vi "Func-엑셀 데이터를 그래프로 출력.vi"() -> ()   [LabVIEW 2015] (continued)
586.53\n586.54\n586.56\n586.58\n586.59\n586.61\n586.63\n586.64\n586.66\n586.68\n586.69\n586.71\n586.73\n586.74\n586.76\n586.78\n586.79\n586.81\n586.83\n586.84\n586.86\n586.88\n586.89\n586.91\n586.93\n586.95\n586.96\n586.98\n586.99\n587.01\n587.03\n587.04\n587.06\n587.08\n587.09\n587.11\n587.13\n587.14\n587.16\n587.18\n587.19\n587.21\n587.23\n587.24\n587.26\n587.28\n587.29\n587.31\n587.33\n587.34\n587.36\n587.38\n587.39\n587.41\n587.43\n587.44\n587.46\n587.48\n587.49\n587.51\n587.53\n587.54\n587.56\n587.58\n587.59\n587.61\n587.63\n587.65\n587.66\n587.68\n587.69\n587.71\n587.73\n587.74\n587.76\n587.78\n587.79\n587.81\n587.83\n587.84\n587.86\n587.88\n587.89\n587.91\n587.93\n587.94\n587.96\n587.98\n587.99\n588.01\n588.03\n588.04\n588.06\n588.08\n588.09\n588.11\n588.13\n588.14\n588.16\n588.18\n588.19\n588.21\n588.23\n588.24\n588.26\n588.28\n588.29\n588.31\n588.33\n588.34\n588.36\n588.38\n588.39\n588.41\n588.43\n588.44\n588.46\n588.48\n588.49\n588.51\n588.53\n588.54\n588.56\n588.58\n588.59\n588.61\n588.63\n588.64\n588.66\n588.68\n588.69\n588.71\n588.73\n588.74\n588.76\n588.78\n588.79\n588.81\n588.83\n588.84\n588.86\n588.88\n588.89\n588.91\n588.93\n588.94\n588.96\n588.98\n589\n589.01\n589.03\n589.04\n589.06\n589.08\n589.09\n589.11\n589.13\n589.14\n589.16\n589.18\n589.19\n589.21\n589.23\n589.24\n589.26\n589.28\n589.29\n589.31\n589.33\n589.35\n589.36\n589.38\n589.39\n589.41\n589.43\n589.45\n589.46\n589.48\n589.49\n589.51\n589.53\n589.54\n589.56\n589.58\n589.6\n589.61\n589.63\n589.64\n589.66\n589.68\n589.69\n589.71\n589.73\n589.74\n589.76\n589.78\n589.79\n589.81\n589.83\n589.84\n589.86\n589.88\n589.89\n589.91\n589.93\n589.94\n589.96\n589.98\n589.99\n590.01\n590.03\n590.04\n590.06\n590.08\n590.09\n590.11\n590.13\n590.15\n590.16\n590.18\n590.19\n590.21\n590.23\n590.24\n590.26\n590.28\n590.29\n590.31\n590.33\n590.34\n590.36\n590.38\n590.39\n590.41\n590.43\n590.44\n590.46\n590.48\n590.5\n590.51\n590.53\n590.54\n590.56\n590.58\n590.59\n590.61\n590.63\n590.64\n590.66\n590.68\n590.69\n590.71\n590.73\n590.74\n590.76\n590.78\n590.79\n590.81\n590.83\n590.84\n590.86\n590.88\n590.89\n590.91\n590.93\n590.94\n590.96\n590.98\n590.99\n591.01\n591.03\n591.04\n591.06\n591.08\n591.09\n591.11\n591.13\n591.14\n591.16\n591.18\n591.19\n591.21\n591.23\n591.24\n591.26\n591.28\n591.29\n591.31\n591.33\n591.34\n591.36\n591.38\n591.39\n591.41\n591.43\n591.44\n591.46\n591.48\n591.49\n591.51\n591.53\n591.54\n591.56\n591.58\n591.59\n591.61\n591.63\n591.64\n591.66\n591.68\n591.69\n591.71\n591.73\n591.75\n591.76\n591.78\n591.79\n591.81\n591.83\n591.84\n591.86\n591.88\n591.89\n591.91\n591.93\n591.94\n591.96\n591.98\n591.99\n592.01\n592.03\n592.04\n592.06\n592.08\n592.1\n592.11\n592.13\n592.14\n592.16\n592.18\n592.19\n592.21\n592.23\n592.24\n592.26\n592.28\n592.29\n592.31\n592.33\n592.34\n592.36\n592.38\n592.39\n592.41\n592.43\n592.45\n592.46\n592.48\n592.49\n592.51\n592.53\n592.54\n592.56\n592.58\n592.59\n592.61\n592.63\n592.64\n592.66\n592.68\n592.7\n592.71\n592.73\n592.74\n592.76\n592.78\n592.8\n592.81\n592.83\n592.84\n592.86\n592.88\n592.89\n592.91\n592.93\n592.94\n592.96\n592.98\n592.99\n593.01\n593.03\n593.05\n593.06\n593.08\n593.09\n593.11\n593.13\n593.15\n593.16\n593.18\n593.19\n593.21\n593.23\n593.25\n593.26\n593.28\n593.29\n593.31\n593.33\n593.34\n593.36\n593.38\n593.39\n593.41\n593.43\n593.44\n593.46\n593.48\n593.49\n593.51\n593.53\n593.54\n593.56\n593.58\n593.59\n593.61\n593.63\n593.65\n593.66\n593.68\n593.69\n593.71\n593.73\n593.75\n593.76\n593.78\n593.79\n593.81\n593.83\n593.84\n593.86\n593.88\n593.89\n593.91\n593.93\n593.94\n593.96\n593.98\n593.99\n594.01\n594.03\n594.04\n594.06\n594.08\n594.09\n594.11\n594.13\n594.14\n594.16\n594.18\n594.19\n594.21\n594.23\n594.24\n594.26\n594.28\n594.29\n594.31\n594.33\n594.34\n594.36\n594.38\n594.39\n594.41\n594.43\n594.44\n594.46\n594.48\n594.49\n594.51\n594.53\n594.54\n594.56\n594.58\n594.59\n594.61\n594.63\n594.64\n594.66\n594.68\n594.69\n594.71\n594.73\n594.74\n594.76\n594.78\n594.79\n594.81\n594.83\n594.85\n594.86\n594.88\n594.89\n594.91\n594.93\n594.94\n594.96\n594.98\n594.99\n595.01\n595.03\n595.04\n595.06\n595.08\n595.09\n595.11\n595.13\n595.14\n595.16\n595.18\n595.2\n595.21\n595.23\n595.24\n595.26\n595.28\n595.29\n595.31\n595.33\n595.34\n595.36\n595.38\n595.39\n595.41\n595.43\n595.45\n595.46\n595.48\n595.49\n595.51\n595.53\n595.55\n595.56\n595.58\n595.59\n595.61\n595.63\n595.64\n595.66\n595.68\n595.69\n595.71\n595.73\n595.74\n595.76\n595.78\n595.8\n595.81\n595.83\n595.84\n595.86\n595.88\n595.89\n595.91\n595.93\n595.94\n595.96\n595.98\n595.99\n596.01\n596.03\n596.04\n596.06\n596.08\n596.09\n596.11\n596.13\n596.14\n596.16\n596.18\n596.19\n596.21\n596.23\n596.24\n596.26\n596.28\n596.29\n596.31\n596.33\n596.34\n596.36\n596.38\n596.39\n596.41\n596.43\n596.44\n596.46\n596.48\n596.5\n596.51\n596.53\n596.54\n596.56\n596.58\n596.6\n596.61\n596.63\n596.64\n596.66\n596.68\n596.7\n596.71\n596.73\n596.74\n596.76\n596.78\n596.79\n596.81\n596.83\n596.84\n596.86\n596.88\n596.89\n596.91\n596.93\n596.94\n596.96\n596.98\n596.99\n597.01\n597.03\n597.04\n597.06\n597.08\n597.09\n597.11\n597.13\n597.14\n597.16\n597.18\n597.19\n597.21\n597.23\n597.24\n597.26\n597.28\n597.29\n597.31\n597.33\n597.34\n597.36\n597.38\n597.39\n597.41\n597.43\n597.44\n597.46\n597.48\n597.49\n597.51\n597.53\n597.54\n597.56\n597.58\n597.59\n597.61\n597.63\n597.64\n597.66\n597.68\n597.69\n597.71\n597.73\n597.74\n597.76\n597.78\n597.79\n597.81\n597.83\n597.84\n597.86\n597.88\n597.89\n597.91\n597.93\n597.94\n597.96\n597.98\n597.99\n598.01\n598.03\n598.04\n598.06\n598.08\n598.09\n598.11\n598.13\n598.14\n598.16\n598.18\n598.2\n598.21\n598.23\n598.24\n598.26\n598.28\n598.29\n598.31\n598.33\n598.34\n598.36\n598.38\n598.39\n598.41\n598.43\n598.44\n598.46\n598.48\n598.49\n598.51\n598.53\n598.55\n598.56\n598.58\n598.59\n598.61\n598.63\n598.65\n598.66\n598.68\n598.69\n598.71\n598.73\n598.74\n598.76\n598.78\n598.8\n598.81\n598.83\n598.84\n598.86\n598.88\n598.9\n598.91\n598.93\n598.94\n598.96\n598.98\n599\n599.01\n599.03\n599.04\n599.06\n599.08\n599.09\n599.11\n599.13\n599.14\n599.16\n599.18\n599.19\n599.21\n599.23\n599.25\n599.26\n599.28\n599.29\n599.31\n599.33\n599.34\n599.36\n599.38\n599.39\n599.41\n599.43\n599.44\n599.46\n599.48\n599.49\n599.51\n599.53\n599.54\n599.56\n599.58\n599.59\n599.61\n599.63\n599.64\n599.66\n599.68\n599.69\n599.71\n599.73\n599.75\n599.76\n599.78\n599.79\n599.81\n599.83\n599.84\n599.86\n599.88\n599.89\n599.91\n599.93\n599.94\n599.96\n599.98\n599.99\n600.01\n600.03\n600.04\n600.06\n600.08\n600.09\n600.11\n600.13\n600.14\n600.16\n600.18\n600.19\n600.21\n600.23\n600.24\n600.26\n600.28\n600.29\n600.31\n600.33\n600.34\n600.36\n600.38\n600.39\n600.41\n600.43\n600.44\n600.46\n600.48\n600.49\n600.51\n600.53\n600.54\n600.56\n600.58\n600.59\n600.61\n600.63\n600.64\n600.66\n600.68\n600.69\n600.71\n600.73\n600.74\n600.76\n600.78\n600.79\n600.81\n600.83\n600.84\n600.86\n600.88\n600.89\n600.91\n600.93\n600.94\n600.96\n600.98\n600.99\n601.01\n601.03\n601.04\n601.06\n601.08\n601.09\n601.11\n601.13\n601.14\n601.16\n601.18\n601.19\n601.21\n601.23\n601.24\n601.26\n601.28\n601.3\n601.31\n601.33\n601.34\n601.36\n601.38\n601.39\n601.41\n601.43\n601.44\n601.46\n601.48\n601.49\n601.51\n601.53\n601.54\n601.56\n601.58\n601.59\n601.61\n601.63\n601.65\n601.66\n601.68\n601.69\n601.71\n601.73\n601.75\n601.76\n601.78\n601.79\n601.81\n601.83\n601.84\n601.86\n601.88\n601.9\n601.91\n601.93\n601.94\n601.96\n601.98\n602\n602.01\n602.03\n602.04\n602.06\n602.08\n602.09\n602.11\n602.13\n602.14\n602.16\n602.18\n602.19\n602.21\n602.23\n602.25\n602.26\n602.28\n602.29\n602.31\n602.33\n602.34\n602.36\n602.38\n602.39\n602.41\n602.43\n602.44\n602.46\n602.48\n602.49\n602.51\n602.53\n602.54\n602.56\n602.58\n602.6\n602.61\n602.63\n602.64\n602.66\n602.68\n602.69\n602.71\n602.73\n602.74\n602.76\n602.78\n602.79\n602.81\n602.83\n602.84\n602.86\n602.88\n602.89\n602.91\n602.93\n602.94\n602.96\n602.98\n602.99\n603.01\n603.03\n603.04\n603.06\n603.08\n603.09\n603.11\n603.13\n603.14\n603.16\n603.18\n603.19\n603.21\n603.23\n603.24\n603.26\n603.28\n603.29\n603.31\n603.33\n603.34\n603.36\n603.38\n603.39\n603.41\n603.43\n603.44\n603.46\n603.48\n603.49\n603.51\n603.53\n603.54\n603.56\n603.58\n603.59\n603.61\n603.63\n603.64\n603.66\n603.68\n603.69\n603.71\n603.73\n603.74\n603.76\n603.78\n603.79\n603.81\n603.83\n603.84\n603.86\n603.88\n603.89\n603.91\n603.93\n603.94\n603.96\n603.98\n603.99\n604.01\n604.03\n604.04\n604.06\n604.08\n604.09\n604.11\n604.13\n604.14\n604.16\n604.18\n604.19\n604.21\n604.23\n604.24\n604.26\n604.28\n604.29\n604.31\n604.33\n604.34\n604.36\n604.38\n604.4\n604.41\n604.43\n604.44\n604.46\n604.48\n604.49\n604.51\n604.53\n604.54\n604.56\n604.58\n604.59\n604.61\n604.63\n604.64\n604.66\n604.68\n604.69\n604.71\n604.73\n604.75\n604.76\n604.78\n604.79\n604.81\n604.83\n604.85\n604.86\n604.88\n604.89\n604.91\n604.93\n604.94\n604.96\n604.98\n605\n605.01\n605.03\n605.04\n605.06\n605.08\n605.1\n605.11\n605.13\n605.14\n605.16\n605.18\n605.19\n605.21\n605.23\n605.24\n605.26\n605.28\n605.29\n605.31\n605.33\n605.34\n605.36\n605.38\n605.39\n605.41\n605.43\n605.44\n605.46\n605.48\n605.49\n605.51\n605.53\n605.55\n605.56\n605.58\n605.59\n605.61\n605.63\n605.64\n605.66\n605.68\n605.69\n605.71\n605.73\n605.74\n605.76\n605.78\n605.8\n605.81\n605.83\n605.84\n605.86\n605.88\n605.89\n605.91\n605.93\n605.94\n605.96\n605.98\n605.99\n606.01\n606.03\n606.04\n606.06\n606.08\n606.09\n606.11\n606.13\n606.14\n606.16\n606.18\n606.19\n606.21\n606.23\n606.24\n606.26\n606.28\n606.29\n606.31\n606.33\n606.34\n606.36\n606.38\n606.39\n606.41\n606.43\n606.44\n606.46\n606.48\n606.49\n606.51\n606.53\n606.54\n606.56\n606.58\n606.59\n606.61\n606.63\n606.64\n606.66\n606.68\n606.69\n606.71\n606.73\n606.74\n606.76\n606.78\n606.79\n606.81\n606.83\n606.84\n606.86\n606.88\n606.89\n606.91\n606.93\n606.94\n606.96\n606.98\n606.99\n607.01\n607.03\n607.04\n607.06\n607.08\n607.09\n607.11\n607.13\n607.14\n607.16\n607.18\n607.19\n607.21\n607.23\n607.24\n607.26\n607.28\n607.29\n607.31\n607.33\n607.34\n607.36\n607.38\n607.39\n607.41\n607.43\n607.44\n607.46\n607.48\n607.5\n607.51\n607.53\n607.54\n607.56\n607.58\n607.59\n607.61\n607.63\n607.64\n607.66\n607.68\n607.69\n607.71\n607.73\n607.75\n607.76\n607.78\n607.79\n607.81\n607.83\n607.85\n607.86\n607.88\n607.89\n607.91\n607.93\n607.94\n607.96\n607.98\n607.99\n608.01\n608.03\n608.04\n608.06\n608.08\n608.09\n608.11\n608.13\n608.14\n608.16\n608.18\n608.19\n608.21\n608.23\n608.24\n608.26\n608.28\n608.29\n608.31\n608.33\n608.34\n608.36\n608.38\n608.39\n608.41\n608.43\n608.44\n608.46\n608.48\n608.49\n608.51\n608.53\n608.55\n608.56\n608.58\n608.59\n608.61\n608.63\n608.64\n608.66\n608.68\n608.69\n608.71\n608.73\n608.74\n608.76\n608.78\n608.8\n608.81\n608.83\n608.84\n608.86\n608.88\n608.89\n608.91\n608.93\n608.94\n608.96\n608.98\n608.99\n609.01\n609.03\n609.04\n609.06\n609.08\n609.09\n609.11\n609.13\n609.14\n609.16\n609.18\n609.19\n609.21\n609.23\n609.24\n609.26\n609.28\n609.29\n609.31\n609.33\n609.34\n609.36\n609.38\n609.39\n609.41\n609.43\n609.44\n609.46\n609.48\n609.49\n609.51\n609.53\n609.54\n609.56\n609.58\n609.59\n609.61\n609.63\n609.64\n609.66\n609.68\n609.69\n609.71\n609.73\n609.74\n609.76\n609.78\n609.79\n609.81\n609.83\n609.84\n609.86\n609.88\n609.89\n609.91\n609.93\n609.94\n609.96\n609.98\n609.99\n610.01\n610.03\n610.04\n610.06\n610.08\n610.09\n610.11\n610.13\n610.14\n610.16\n610.18\n610.19\n610.21\n610.23\n610.24\n610.26\n610.28\n610.29\n610.31\n610.33\n610.34\n610.36\n610.38\n610.39\n610.41\n610.43\n610.44\n610.46\n610.48\n610.5\n610.51\n610.53\n610.54\n610.56\n610.58\n610.6\n610.61\n610.63\n610.64\n610.66\n610.68\n610.69\n610.71\n610.73\n610.74\n610.76\n610.78\n610.79\n610.81\n610.83\n610.85\n610.86\n610.88\n610.89\n610.91\n610.93\n610.95\n610.96\n610.98\n610.99\n611.01\n611.03\n611.04\n611.06\n611.08\n611.1\n611.11\n611.13\n611.14\n611.16\n611.18\n611.2\n611.21\n611.23\n611.24\n611.26\n611.28\n611.3\n611.31\n611.33\n611.34\n611.36\n611.38\n611.39\n611.41\n611.43\n611.44\n611.46\n611.48\n611.49\n611.51\n611.53\n611.54\n611.56\n611.58\n611.59\n611.61\n611.63\n611.64\n611.66\n611.68\n611.69\n611.71\n611.73\n611.74\n611.76\n611.78\n611.79\n611.81\n611.83\n611.84\n611.86\n611.88\n611.89\n611.91\n611.93\n611.94\n611.96\n611.98\n611.99\n612.01\n612.03\n612.04\n612.06\n612.08\n612.09\n612.11\n612.13\n612.14\n612.16\n612.18\n612.19\n612.21\n612.23\n612.24\n612.26\n612.28\n612.29\n612.31\n612.33\n612.35\n612.36\n612.38\n612.39\n612.41\n612.43\n612.44\n612.46\n612.48\n612.49\n612.51\n612.53\n612.54\n612.56\n612.58\n612.59\n612.61\n612.63\n612.64\n612.66\n612.68\n612.69\n612.71\n612.73\n612.74\n612.76\n612.78\n612.79\n612.81\n612.83\n612.84\n612.86\n612.88\n612.89\n612.91\n612.93\n612.94\n612.96\n612.98\n612.99\n613.01\n613.03\n613.04\n613.06\n613.08\n613.09\n613.11\n613.13\n613.14\n613.16\n613.18\n613.19\n613.21\n613.23\n613.24\n613.26\n613.28\n613.29\n613.31\n613.33\n613.34\n613.36\n613.38\n613.39\n613.41\n613.43\n613.44\n613.46\n613.48\n613.49\n613.51\n613.53\n613.54\n613.56\n613.58\n613.6\n613.61\n613.63\n613.64\n613.66\n613.68\n613.69\n613.71\n613.73\n613.74\n613.76\n613.78\n613.79\n613.81\n613.83\n613.84\n613.86\n613.88\n613.89\n613.91\n613.93\n613.95\n613.96\n613.98\n613.99\n614.01\n614.03\n614.04\n614.06\n614.08\n614.09\n614.11\n614.13\n614.14\n614.16\n614.18\n614.2\n614.21\n614.23\n614.24\n614.26\n614.28\n614.29\n614.31\n614.33\n614.34\n614.36\n614.38\n614.39\n614.41\n614.43\n614.45\n614.46\n614.48\n614.49\n614.51\n614.53\n614.55\n614.56\n614.58\n614.59\n614.61\n614.63\n614.64\n614.66\n614.68\n614.69\n614.71\n614.73\n614.74\n614.76\n614.78\n614.79\n614.81\n614.83\n614.84\n614.86\n614.88\n614.9\n614.91\n614.93\n614.94\n614.96\n614.98\n614.99\n615.01\n615.03\n615.04\n615.06\n615.08\n615.1\n615.11\n615.13\n615.14\n615.16\n615.18\n615.19\n615.21\n615.23\n615.24\n615.26\n615.28\n615.29\n615.31\n615.33\n615.34\n615.36\n615.38\n615.39\n615.41\n615.43\n615.44\n615.46\n615.48\n615.49\n615.51\n615.53\n615.54\n615.56\n615.58\n615.59\n615.61\n615.63\n615.64\n615.66\n615.68\n615.69\n615.71\n615.73\n615.74\n615.76\n615.78\n615.79\n615.81\n615.83\n615.84\n615.86\n615.88\n615.89\n615.91\n615.93\n615.94\n615.96\n615.98\n615.99\n616.01\n616.03\n616.04\n616.06\n616.08\n616.09\n616.11\n616.13\n616.14\n616.16\n616.18\n616.19\n616.21\n616.23\n616.24\n616.26\n616.28\n616.29\n616.31\n616.33\n616.35\n616.36\n616.38\n616.39\n616.41\n616.43\n616.44\n616.46\n616.48\n616.49\n616.51\n616.53\n616.54\n616.56\n616.58\n616.59\n616.61\n616.63\n616.64\n616.66\n616.68\n616.7\n616.71\n616.73\n616.74\n616.76\n616.78\n616.79\n616.81\n616.83\n616.84\n616.86\n616.88\n616.89\n616.91\n616.93\n616.94\n616.96\n616.98\n616.99\n617.01\n617.03\n617.05\n617.06\n617.08\n617.09\n617.11\n617.13\n617.14\n617.16\n617.18\n617.19\n617.21\n617.23\n617.24\n617.26\n617.28\n617.3\n617.31\n617.33\n617.34\n617.36\n617.38\n617.4\n617.41\n617.43\n617.44\n617.46\n617.48\n617.49\n617.51\n617.53\n617.54\n617.56\n617.58\n617.59\n617.61\n617.63\n617.65\n617.66\n617.68\n617.69\n617.71\n617.73\n617.74\n617.76\n617.78\n617.79\n617.81\n617.83\n617.84\n617.86\n617.88\n617.89\n617.91\n617.93\n617.94\n617.96\n617.98\n617.99\n618.01\n618.03\n618.04\n618.06\n618.08\n618.09\n618.11\n618.13\n618.14\n618.16\n618.18\n618.19\n618.21\n618.23\n618.24\n618.26\n618.28\n618.29\n618.31\n618.33\n618.34\n618.36\n618.38\n618.39\n618.41\n618.43\n618.44\n618.46\n618.48\n618.49\n618.51\n618.53\n618.54\n618.56\n618.58\n618.59\n618.61\n618.63\n618.64\n618.66\n618.68\n618.69\n618.71\n618.73\n618.74\n618.76\n618.78\n618.79\n618.81\n618.83\n618.84\n618.86\n618.88\n618.89\n618.91\n618.93\n618.94\n618.96\n618.98\n618.99\n619.01\n619.03\n619.04\n619.06\n619.08\n619.09\n619.11\n619.13\n619.14\n619.16\n619.18\n619.19\n619.21\n619.23\n619.24\n619.26\n619.28\n619.29\n619.31\n619.33\n619.34\n619.36\n619.38\n619.39\n619.41\n619.43\n619.45\n619.46\n619.48\n619.49\n619.51\n619.53\n619.54\n619.56\n619.58\n619.59\n619.61\n619.63\n619.64\n619.66\n619.68\n619.69\n619.71\n619.73\n619.74\n619.76\n619.78\n619.8\n619.81\n619.83\n619.84\n619.86\n619.88\n619.89\n619.91\n619.93\n619.94\n619.96\n619.98\n619.99\n620.01\n620.03\n620.05\n620.06\n620.08\n620.09\n620.11\n620.13\n620.15\n620.16\n620.18\n620.19\n620.21\n620.23\n620.25\n620.26\n620.28\n620.29\n620.31\n620.33\n620.34\n620.36\n620.38\n620.4\n620.41\n620.43\n620.44\n620.46\n620.48\n620.5\n620.51\n620.53\n620.54\n620.56\n620.58\n620.59\n620.61\n620.63\n620.65\n620.66\n620.68\n620.69\n620.71\n620.73\n620.74\n620.76\n620.78\n620.79\n620.81\n620.83\n620.84\n620.86\n620.88\n620.89\n620.91\n620.93\n620.95\n620.96\n620.98\n621\n621.01\n621.03\n621.04\n621.06\n621.08\n621.09\n621.11\n621.13\n621.14\n621.16\n621.18\n621.19\n621.21\n621.23\n621.24\n621.26\n621.28\n621.29\n621.31\n621.33\n621.34\n621.36\n621.38\n621.39\n621.41\n621.43\n621.44\n621.46\n621.48\n621.49\n621.51\n621.53\n621.54\n621.56\n621.58\n621.59\n621.61\n621.63\n621.64\n621.66\n621.68\n621.69\n621.71\n621.73\n621.74\n621.76\n621.78\n621.79\n621.81\n621.83\n621.84\n621.86\n621.88\n621.89\n621.91\n621.93\n621.94\n621.96\n621.98\n621.99\n622.01\n622.03\n622.04\n622.06\n622.08\n622.09\n622.11\n622.13\n622.14\n622.16\n622.18\n622.19\n622.21\n622.23\n622.24\n622.26\n622.28\n622.29\n622.31\n622.33\n622.34\n622.36\n622.38\n622.39\n622.41\n622.43\n622.44\n622.46\n622.48\n622.49\n622.51\n622.53\n622.54\n622.56\n622.58\n622.59\n622.61\n622.63\n622.64\n622.66\n622.68\n622.69\n639.46\n639.62\n639.63\n639.64\n639.66\n639.68\n639.69\n639.71\n639.73\n639.74\n639.76\n639.78\n639.79\n639.81\n639.83\n639.84\n639.86\n639.88\n639.89\n639.91\n639.93\n639.94\n639.96\n639.98\n639.99\n640.01\n640.03\n640.04\n640.06\n640.08\n640.09\n640.11\n640.13\n640.14\n640.16\n640.18\n640.19\n640.21\n640.23\n640.24\n640.26\n640.28\n640.29\n640.31\n640.33\n640.35\n640.36\n640.38\n640.39\n640.41\n640.43\n640.44\n640.46\n640.48\n640.49\n640.51\n640.53\n640.54\n640.56\n640.58\n640.59\n640.61\n640.63\n640.64\n640.66\n640.68\n640.7\n640.71\n640.73\n640.74\n640.76\n640.78\n640.79\n640.81\n640.83\n640.84\n640.86\n640.88\n640.89\n640.91\n640.93\n640.95\n640.96\n640.98\n640.99\n641.01\n641.03\n641.05\n641.06\n641.08\n641.09\n641.11\n641.13\n641.14\n641.16\n641.18\n641.19\n641.21\n641.23\n641.24\n641.26\n641.28\n641.3\n641.31\n641.33\n641.34\n641.36\n641.38\n641.4\n641.41\n641.43\n641.44\n641.46\n641.48\n641.49\n641.51\n641.53\n641.54\n641.56\n641.58\n641.59\n641.61\n641.63\n641.64\n641.66\n641.68\n641.69\n641.71\n641.73\n641.74\n641.76\n641.78\n641.79\n641.81\n641.83\n641.84\n641.86\n641.88\n641.89\n641.91\n641.93\n641.94\n641.96\n641.98\n642\n642.01\n642.03\n642.04\n642.06\n642.08\n642.09\n642.11\n642.13\n642.14\n642.16\n642.18\n642.19\n642.21\n642.23\n642.24\n642.26\n642.28\n642.29\n642.31\n642.33\n642.34\n642.36\n642.38\n642.39\n642.41\n642.43\n642.44\n642.46\n642.48\n642.49\n642.51\n642.53\n642.54\n642.56\n642.58\n642.59\n642.61\n642.63\n642.64\n642.66\n642.68\n642.69\n642.71\n642.73\n642.74\n642.76\n642.78\n642.79\n642.81\n642.83\n642.84\n642.86\n642.88\n642.89\n642.91\n642.93\n642.94\n642.96\n642.98\n642.99\n643.01\n643.03\n643.04\n643.06\n643.08\n643.09\n643.11\n643.13\n643.14\n643.16\n643.18\n643.19\n643.21\n643.23\n643.24\n643.26\n643.28\n643.29\n643.31\n643.33\n643.34\n643.36\n643.38\n643.39\n643.41\n643.43\n643.44\n643.46\n643.48\n643.49\n643.51\n643.53\n643.54\n643.56\n643.58\n643.59\n643.61\n643.63\n643.64\n643.66\n643.68\n643.69\n643.71\n643.73\n643.74\n643.76\n643.78\n643.79\n643.81\n643.83\n643.84\n643.86\n643.88\n643.89\n643.91\n643.93\n643.94\n643.96\n643.98\n643.99\n644.01\n644.03\n644.05\n644.06\n644.08\n644.09\n644.11\n644.13\n644.15\n644.16\n644.18\n644.19\n644.21\n644.23\n644.24\n644.26\n644.28\n644.29\n644.31\n644.33\n644.34\n644.36\n644.38\n644.4\n644.41\n644.43\n644.44\n644.46\n644.48\n644.5\n644.51\n644.53\n644.54\n644.56\n644.58\n644.59\n644.61\n644.63\n644.64\n644.66\n644.68\n644.69\n644.71\n644.73\n644.74\n644.76\n644.78\n644.79\n644.81\n644.83\n644.85\n644.86\n644.88\n644.89\n644.91\n644.93\n644.94\n644.96\n644.98\n644.99\n645.01\n645.03\n645.04\n645.06\n645.08\n645.09\n645.11\n645.13\n645.14\n645.16\n645.18\n645.19\n
